vi "Remove XLSX Empty Columns.vi"(8 "error in (no error)":errorcluster, 11 "Array in":string[][](array[string])) -> (0 "error out":errorcluster, 1 "Removed Column Indices":i32[](array[numeric]), 3 "Array out":string[][](array[string]))   [LabVIEW 2021, in "Files.lvlib"]
doc: "Fills table with copies of the single-copy value of multicell-spanning super-cell."
uses:
  Files.lvlib
panel:
  # "see the AlliGator License on the block diagram (Ctrl+E or Window:Show Block Diagram)"
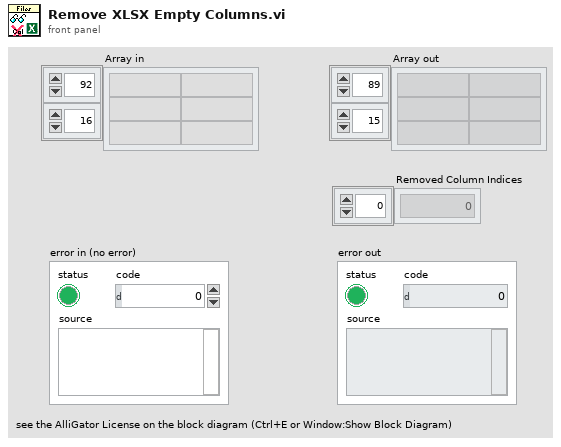
[diagram p1: front panel]
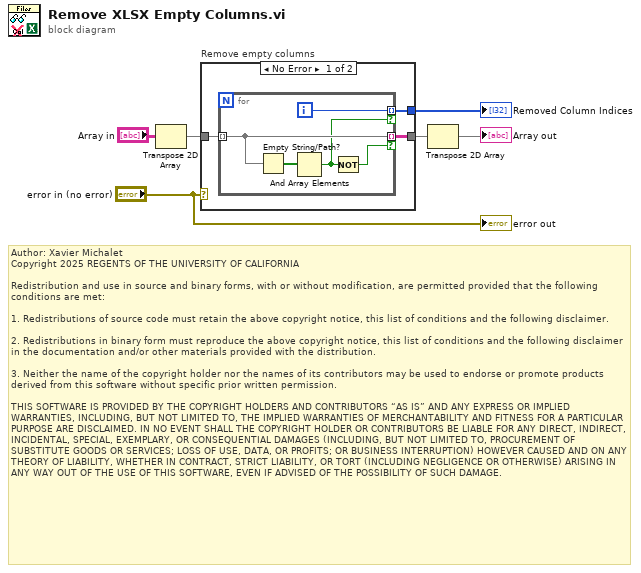
[diagram p0: block diagram]
diagram:
  # "Author: Xavier Michalet\nCopyright 2025 REGENTS OF THE UNIVERSITY OF CALIFORNIA\n\nRedistribution and use in source and binary forms, with or without modification, are permitted provided that the following conditions are met:\n\n1. Redistributions of source code must retain the above copyright notice, this list of conditions and the following disclaimer.\n\n2. Redistributions in binary form must reproduce the above copyright notice, this list of conditions and the following disclaimer in the documentation and/or other materials provided with the distribution.\n\n3. Neither the name of the copyright holder nor the names of its contributors may be used to endorse or promote products derived from this software without specific prior written permission.\n\nTHIS SOFTWARE IS PROVIDED BY THE COPYRIGHT HOLDERS AND CONTRIBUTORS “AS IS” AND ANY EXPRESS OR IMPLIED WARRANTIES, INCLUDING, BUT NOT LIMITED TO, THE IMPLIED WARRANTIES OF MERCHANTABILITY AND FITNESS FOR A PARTICULAR PURPOSE ARE DISCLAIMED. IN NO EVENT SHALL THE COPYRIGHT HOLDER OR CONTRIBUTORS BE LIABLE FOR ANY DIRECT, INDIRECT, INCIDENTAL, SPECIAL, EXEMPLARY, OR CONSEQUENTIAL DAMAGES (INCLUDING, BUT NOT LIMITED TO, PROCUREMENT OF SUBSTITUTE GOODS OR SERVICES; LOSS OF USE, DATA, OR PROFITS; OR BUSINESS INTERRUPTION) HOWEVER CAUSED AND ON ANY THEORY OF LIABILITY, WHETHER IN CONTRACT, STRICT LIABILITY, OR TORT (INCLUDING NEGLIGENCE OR OTHERWISE) ARISING IN ANY WAY OUT OF THE USE OF THIS SOFTWARE, EVEN IF ADVISED OF THE POSSIBILITY OF SUCH DAMAGE."
  n1 = Transpose 2D Array(2D array="Array in") -> (transposed array=w3:string[][])
  n2 = case "Remove empty columns" shown="No Error" "error in (no error)" {
    tunnel: w3 -> [w9 w15]
    tunnel: [w8 w15] -> w5
    tunnel: [w7 _] -> w1
    frame No Error {
      n3 = for {
        tunnel: w9 -> [w13] mode=indexing
        tunnel: [w13] -> w8 mode=indexing if=w11
        tunnel: [w12] -> w7 mode=indexing if=w10
        i -> [w12]
        n4 = Empty String/Path?(string/path=w13) -> (empty?=w14:bool[])
        n5 = And Array Elements(Boolean array=w14) -> (logical AND=w10:bool)
        n6 = Not(x=w10) -> (.not. x?=w11:bool)
      }
    }
    frame Error {
    }
  }
  "Removed Column Indices" <- w1
  n7 = Transpose 2D Array(2D array=w5) -> (transposed array=→"Array out":string[][])
  "error out" <- "error in (no error)"
